vi "MesGetALLProduct.vi"(6 "equipment_code":string="102", 8 "error in":errorcluster, 10 "类型":string, 11 "connection reference":T1) -> (0 "error out":errorcluster, 1 "查找的结果":string[][](array[string]), 2 "connection out":T1, 3 "错误状态":bool, 5 "非空":bool)   [LabVIEW 2014]
uses:
  <vilib>/addons/database/Connection.llb/Conn ObjectReference.ctl
  <vilib>/addons/database/Connection.llb/DB Tools Open Connec (String).vi
  <vilib>/addons/database/Connection.llb/Conn Execute.vi
  <vilib>/addons/database/Recordset.llb/Rec Fetch Recordset Data (R).vi
  <vilib>/addons/database/Recordset.llb/Rec Destroy - Connection.vi
  <vilib>/addons/database/_DB Variant To Data/Database Variant To Data.xnode
  <vilib>/addons/database/NI_Database_API.lvlib
panel:
  out "SQL_在指定表中指定字段插入数据":string
  out "recordset data":variant[][](array[variant])
  in  "设备编号":string
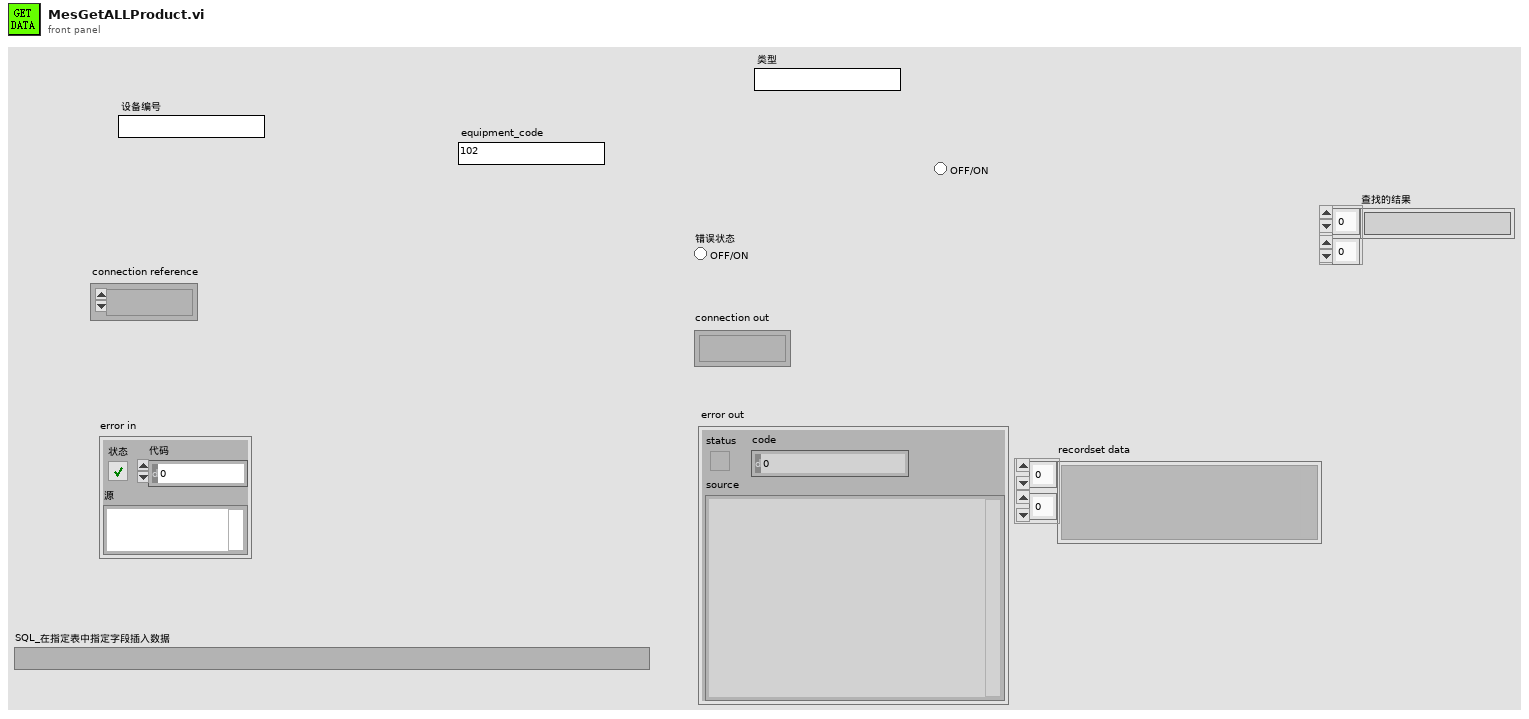
[diagram p1: front panel]
types:
  T1 = typedef "NI_Database_API.lvlib/Conn ObjectReference.ctl" = refnum<k1>
  T2 = typedef "NI_Database_API.lvlib/Rec ObjectReference.ctl" = refnum<k1>
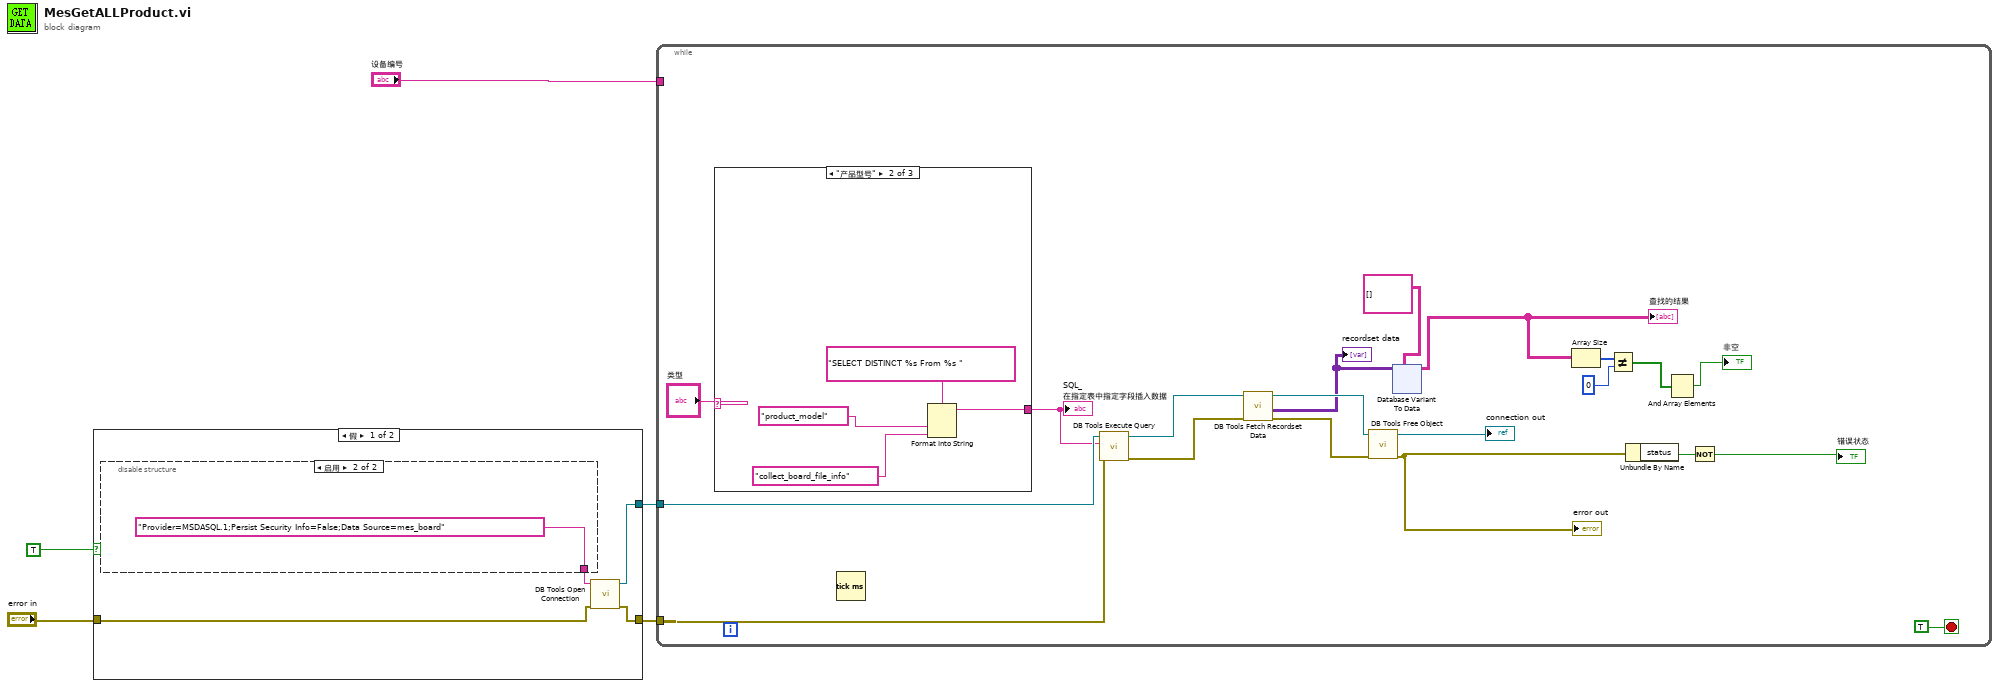
[diagram p0: block diagram]
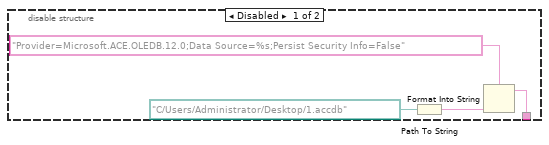
[diagram p2: hidden frame]
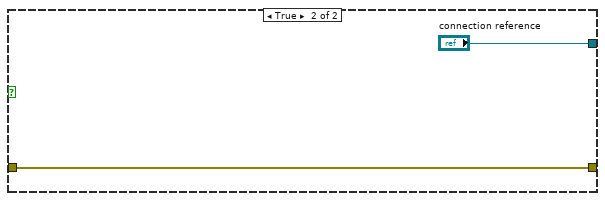
[diagram p3: hidden frame]
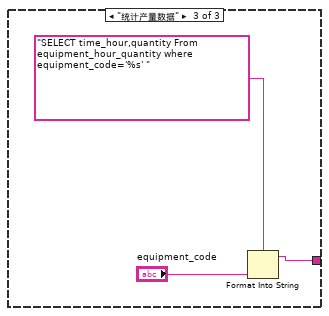
[diagram p5: hidden frame]
diagram:
  n1 = case shown="假" TRUE {
    tunnel: [w9 "connection reference"] -> w2
    tunnel: [w8 w15] -> w3
    tunnel: "error in" -> [w6 w15]
    frame False {
      n2 = disable-structure shown="启用" {
        disable-tunnel: [w12 "Provider=MSDASQL.1;Persist Security Info=False;Data Source=mes_board" ("connection information")] -> w7
        frame Disabled {
          n3 = Path To String(path=path "C:/Users/Administrator/Desktop/1.accdb" ("路径")) -> (string=w13:string)
          n4 = Format Into String(format string="Provider=Microsoft.ACE.OLEDB.12.0;Data Source=%s;Persist Security Info=False" ("初始字符串"), w13) -> (resulting string=w12:string)  [unwired: 2 in, 1 out]
        }
        frame Enabled {
        }
      }
      n5 = call-poly <vilib>:"DB Tools Open Connection.vi"("error in (no error)"=w6, "connection information"=w7) -> ("error out"=w8:errorcluster, "connection reference"=w9:T1)  [unwired: 6 in]
    }
    frame True {
    }
  }
  n6 = while {
    tunnel: w2 -> [w36]
    tunnel: "设备编号" -> [_]
    tunnel: w3 -> [w32]
    stop <- TRUE stop-if-true
    n7 = case shown="\"产品型号\"" "类型" {
      tunnel: [_ w37 w41] -> w24
      frame Default {
      }
      frame "产品型号" {
        n8 = Format Into String(format string="SELECT DISTINCT %s From %s ", "product_model" ("productModel"), "collect_board_file_info" ("表名")) -> (resulting string=w37:string)  [unwired: 2 in, 1 out]
      }
      frame "统计产量数据" {
        n9 = Format Into String(format string="SELECT time_hour,quantity From equipment_hour_quantity where equipment_code='%s' " ("字符串"), "equipment_code") -> (resulting string=w41:string)  [unwired: 2 in, 1 out]
      }
    }
    "SQL_在指定表中指定字段插入数据" <- w24
    n10 = Tick Count (ms)() -> ()  [unwired: 1 out]
    n11 = call-poly <vilib>:"DB Tools Execute Query.vi"("error in (no error)"=w32, "SQL query"=w24, "connection reference"=w36) -> ("error out"=w30:errorcluster, "recordset reference"=w25:T2)  [unwired: 5 in]
    n12 = call-poly <vilib>:"DB Tools Fetch Recordset Data.vi"("error in (no error)"=w30, "recordset reference"=w25) -> ("error out"=w29:errorcluster, "recordset data"=w27:variant[][], "recordset reference out"=w28:T2)  [unwired: 3 in]
    "recordset data" <- w27
    n13 = call-poly <vilib>:"DB Tools Free Object.vi"("error in (no error)"=w29, "recordset reference"=w28) -> ("error out"=w35:errorcluster, "connection reference"=→"connection out":T1)  [unwired: 8 in]
    "error out" <- w35
    n14 = xnode "Database Variant To Data"("database variant"=w27, "type"=string[][] [] ("columns")) -> ("data"=w22:string[][])  [unwired: 1 in, 1 out]
    "查找的结果" <- w22
    n15 = Array Size(array=w22) -> (size(s)=w21:i32[])
    n16 = Not Equal?(x=w21, y=0) -> (x != y?=w20:bool[])
    n17 = Unbundle By Name(w35) -> ("status"=w34:bool)
    n18 = And Array Elements(Boolean array=w20) -> (logical AND=→"非空":bool)
    n19 = Not(x=w34) -> (.not. x?=→"错误状态":bool)
  }
